vi "fgv_tcp_ntrip-client.vi"(7 "cmd":T1, 8 "error in":errorcluster, 9 "w-data":string, 10 "remote port":u16=2101, 11 "address":string="gnss.eseoul.go.kr") -> (0 "error out":errorcluster, 3 "r-data":string)   [LabVIEW 2019]
uses:
  Ctrl/comm-ini-rw-close.ctl
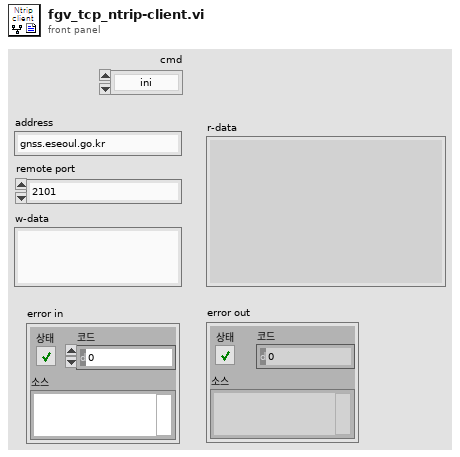
[diagram p1: front panel]
types:
  T1 = typedef "comm-ini-rw-close.ctl" = enum16{"ini", "write", "read", "close"}
  T2 = enum16{"Standard", "Buffered", "CRLF", "Immediate"}
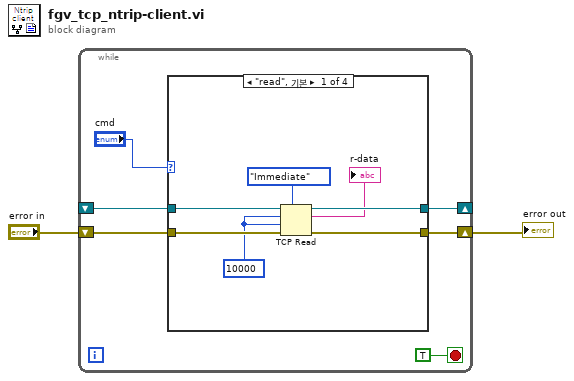
[diagram p0: block diagram]
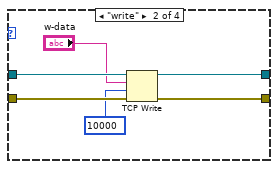
[diagram p2: hidden frame]
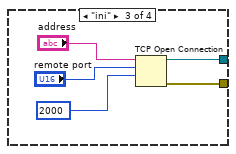
[diagram p3: hidden frame]
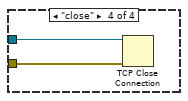
[diagram p4: hidden frame]
diagram:
  n1 = while {
    shift-right: [w7] -> _
    shift-left: _ -> [w5]
    shift-right: [w6] -> w2
    shift-left: "error in" -> [w4]
    stop <- TRUE stop-if-true
    n2 = case shown="\"read\", 기본" "cmd" {
      tunnel: [w15 w20 w23 _] -> w7
      tunnel: [w13 w18 w22 _] -> w6
      tunnel: w5 -> [w12 w21 _ w28]
      tunnel: w4 -> [w14 w19 _ w27]
      frame "read", Default {
        w9 = 10000 ("읽을 바이트")
        n3 = TCP Read(connection ID=w12, bytes to read=w9, error in (no error)=w14, 7:T2."Immediate" ("mode (standard)"), 9:w9) -> (connection ID out=w15:refnum<k5>, data out=→"r-data":string, error out=w13:errorcluster)
      }
      frame "write" {
        n4 = TCP Write(connection ID=w21, data in="w-data", error in (no error)=w19, 9:10000 ("타임아웃 ms (25000)")) -> (connection ID out=w20:refnum<k5>, error out=w18:errorcluster)  [unwired: 1 out]
      }
      frame "ini" {
        n5 = TCP Open Connection(address="address", remote port or service name="remote port", timeout ms (60000)=2000) -> (connection ID=w23:refnum<k5>, error out=w22:errorcluster)  [unwired: 2 in]
      }
      frame "close" {
        n6 = TCP Close Connection(connection ID=w28, error in (no error)=w27) -> ()  [unwired: 1 in, 2 out]
      }
    }
  }
  "error out" <- w2
